vi "H036 Harsh Pandit SCADA Lab 2b Sem 6.vi"() -> ()   [LabVIEW 2018]
panel:
  in  "MSB":bool
  out "Number":dbl
  in  "LSB":bool
  in  "Bit 2":bool
  in  "Bit 3":bool
  # "Experiment 2b: Develope a HMI to convert 4 bit binary number to decimal number"
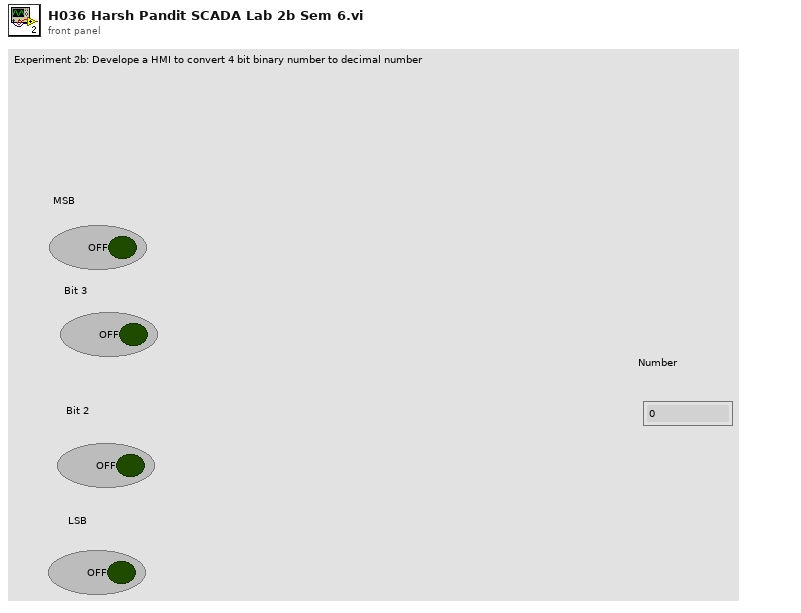
[diagram p1: front panel]
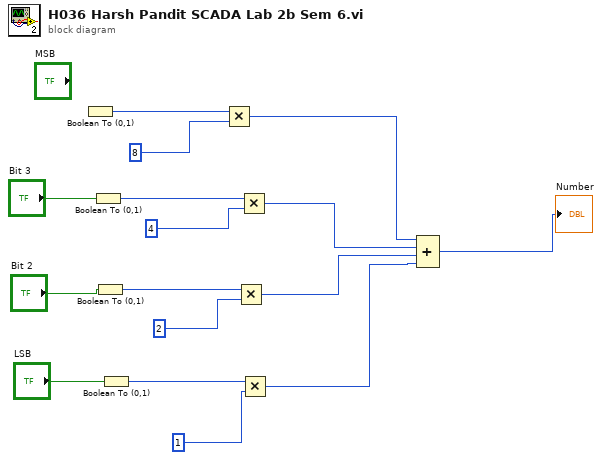
[diagram p0: block diagram]
diagram:
  n1 = Boolean To (0,1)() -> (Boolean=w17:bool, 0, 1=w16:i16)
  n2 = Boolean To (0,1)(Boolean="Bit 3") -> (0, 1=w12:i16)
  n3 = Boolean To (0,1)(Boolean="Bit 2") -> (0, 1=w11:i16)
  n4 = Boolean To (0,1)(Boolean="LSB") -> (0, 1=w10:i16)
  n5 = Multiply(x=w16, y=8) -> (x*y=w9:i32)
  n6 = Multiply(x=w11, y=2) -> (x*y=w7:i32)
  n7 = Multiply(x=w12, y=4) -> (x*y=w8:i32)
  n8 = Multiply(x=w10, y=1) -> (x*y=w6:i32)
  n9 = Compound Arithmetic op=ADD(w9, w8, w7, w6) -> (→"Number":i32)
